vi "brc_daq_disconnect_module.vi"(0 "index":i32, 5 "error in (no error)":errorcluster, 6 "mHandle":i32) -> (19 "error out":errorcluster)   [LabVIEW 2015, in "BRC-DAQ x64.lvlib"]
uses:
  BRC-DAQ x64.lvlib
  DLL/brc_daq_sdk.dll
panel:
  out "return_value":i32
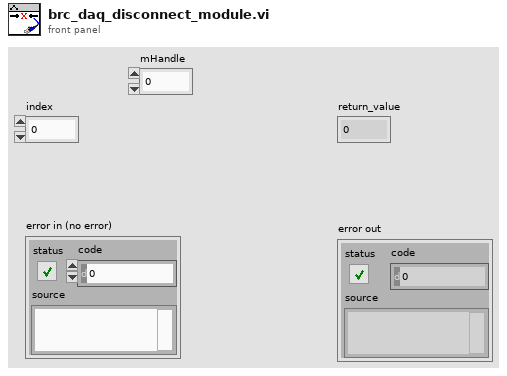
[diagram p1: front panel]
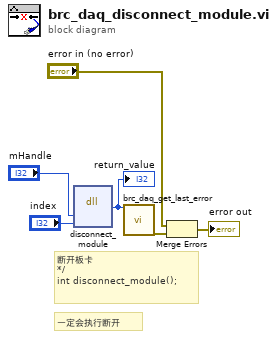
[diagram p0: block diagram]
diagram:
  # "断开板卡\n*/\nint disconnect_module();"
  # "一定会执行断开"
  n1 = dll-call lib="E:/01 BRC project/04BRC-daq/04 Drive/BRC-DAQ/DAQ-x64/DLL/brc_daq_sdk.dll" fn="disconnect_module"("mHandle"="mHandle", "index"="index") -> ("return type"=w3:i32)  [unwired: 5 in, 2 out]
  "return_value" <- w3
  n2 = call "brc_daq_get_last_error.vi"("return_value"=w3) -> ("error out"=w2:errorcluster)  [unwired: 18 in]
  n3 = Merge Errors("error in (no error)", w2) -> (→"error out":errorcluster)
